vi "Dispose.vi"(8 "error in (no error)":errorcluster, 11 "CreatorA":refnum<class "CreatorA.lvclass">) -> (0 "error out":errorcluster)   [LabVIEW 2020, in "FactoryMethod.lvlib" / "FactoryMethodLazyEvaluation.lvlib" / "CreatorA.lvclass"]
uses:
  CreatorA.lvclass
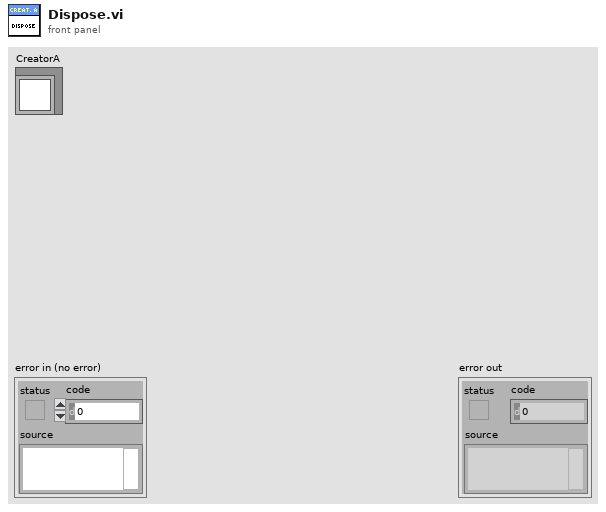
[diagram p1: front panel]
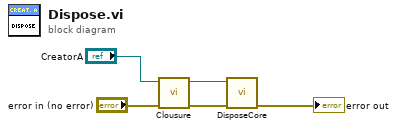
[diagram p0: block diagram]
diagram:
  n1 = call-dynamic "Clousure.vi"("error in (no error)"="error in (no error)", "CreatorA"="CreatorA") -> ("error out"=w3:errorcluster, "CreatorA"=w2:refnum<class "CreatorA.lvclass">)  [unwired: 8 in]
  n2 = call-dynamic "DisposeCore.vi"("error in (no error)"=w3, "CreatorA"=w2) -> ("error out"=→"error out":errorcluster)  [unwired: 8 in, 1 out]
